vi "Cleanup.vi"(8 "error in (no error)":errorcluster) -> (0 "error out":errorcluster)   [LabVIEW 2015, in "Front Panel Publisher.lvlib"]
doc: "This VI closes all sessions and stops execution of any asynchronous processes involved in the web page generation."
uses:
  Front Panel Publisher.lvlib
  Web Front Panel_class/Web Front Panel.lvclass
  Websocket_class/Websocket.lvclass
  Front Panel Manager_class/Front Panel Manager.lvclass
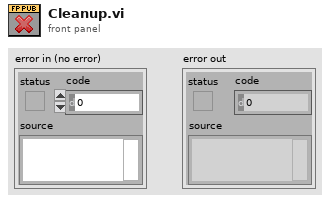
[diagram p1: front panel]
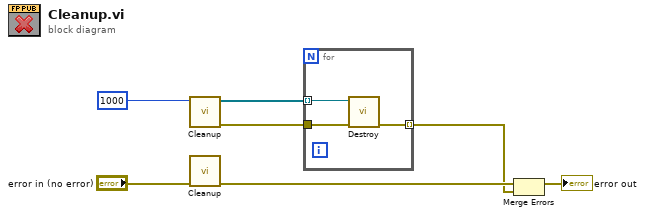
[diagram p0: block diagram]
diagram:
  n1 = call "Cleanup.vi"("Timeout (-1)"=1000 ("ms timeout (-1)")) -> ("error out"=w2:errorcluster, "WebFrontPanels"=w6:refnum<class "Web Front Panel.lvclass">[])  [unwired: 9 in]
  n2 = call "Cleanup.vi"("error in (no error)"="error in (no error)") -> ("error out"=w4:errorcluster)  [unwired: 10 in]
  n3 = for {
    tunnel: w6 -> [w10] mode=indexing
    tunnel: w2 -> [w9]
    tunnel: [w8] -> w1 mode=indexing
    n4 = call-dynamic "Destroy.vi"("error in (no error)"=w9, "Web FP In"=w10) -> ("error out"=w8:errorcluster)  [unwired: 8 in, 1 out]
  }
  n5 = Merge Errors(w4, w1) -> (→"error out":errorcluster)
